vi "Loader Delay.vi"(11 "Input":bool) -> (3 "Position":T1)   [LabVIEW 2012]
uses:
  <vilib>/Rock Robotics/WPI/Relay/WPI_RelayValue.ctl
panel:
  out "Running":bool
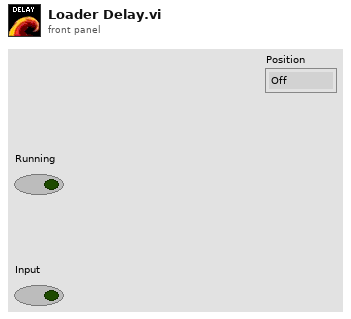
[diagram p1: front panel]
types:
  T1 = typedef "WPI_RelayValue.ctl" = enum16{"Off", "On", "Forward", "Reverse"}
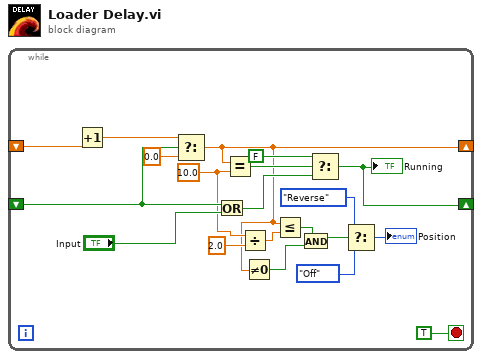
[diagram p0: block diagram]
diagram:
  n1 = while {
    shift-right: [w3] -> _
    shift-left: _ -> [w18]
    shift-right: [w15] -> _
    shift-left: _ -> [w13]
    stop <- TRUE stop-if-true
    w5 = 10.0 ("Times to Run")
    n2 = Increment(x=w18) -> (x+1=w17:dbl)
    n3 = Select(t=w17, s=w13, f=0.0) -> (s? t:f=w3:dbl)
    n4 = Or(x=w13, y="Input") -> (x .or. y?=w12:bool)
    n5 = Equal?(x=w3, y=w5) -> (x = y?=w16:bool)
    n6 = Divide(x=w5, y=2.0) -> (x/y=w9:dbl)
    n7 = Not Equal To 0?(x=w3) -> (x != 0?=w4:bool)
    n8 = Less Or Equal?(x=w3, y=w9) -> (x <= y?=w8:bool)
    n9 = And(x=w8, y=w4) -> (x .and. y?=w6:bool)
    n10 = Select(t=FALSE, s=w16, f=w12) -> (s? t:f=w15:bool)
    "Running" <- w15
    n11 = Select(t=WPI_RelayValue."Reverse" ("RelayValue"), s=w6, f=WPI_RelayValue."Off" ("RelayValue")) -> (s? t:f=→"Position":T1)
  }
